vi "Switch status IO - Human Readable.vi"(1 "Switch status":path=path "C:/LabView/PPMS basic VIs/Switch Status.txt") -> (0 "String":string)   [LabVIEW 2016, in "pickering.lvclass"]
uses:
  pickering.lvclass
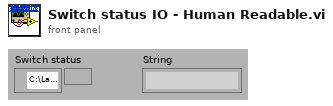
[diagram p1: front panel]
types:
  T1 = typedef "pickering.lvclass/Channels-Array.ctl" = T2[]
  T2 = typedef "pickering.lvclass/Channel-Cluster.ctl" = cluster{"Channel x":T3, "Channel y":T4}
  T3 = typedef "pickering.lvclass/ChannelX-ComboBox.ctl" = string
  T4 = typedef "pickering.lvclass/ChannelY-ComboBox.ctl" = string
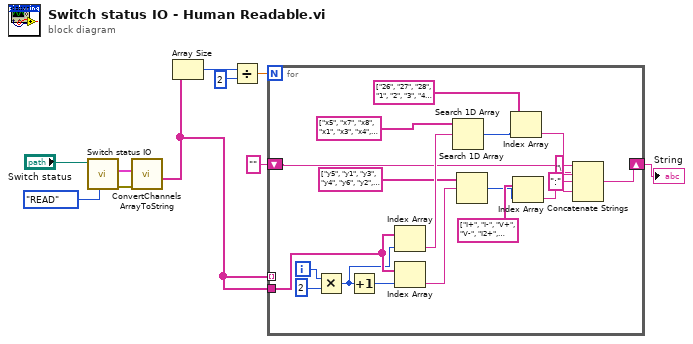
[diagram p0: block diagram]
diagram:
  n1 = call "Switch status IO.vi"("mode"=enum16{"READ", "WRITE"}."READ", "Path"="Switch status") -> ("error out"=w3:errorcluster, "Channels out"=w2:T1)  [unwired: 7 in, 1 out]
  n2 = call "ConvertChannelsArrayToString.vi"("error in (no error)"=w3, "Channels in"=w2) -> ("String array"=w1:string[])  [unwired: 7 in, 2 out]
  n3 = Array Size(array=w1) -> (size(s)=w6:i32)
  n4 = Divide(x=w6, y=2) -> (x/y=w8:dbl)
  n5 = for {
    N: w8 -> [_]
    tunnel: w1 -> [w29]
    tunnel: w1 -> [_] mode=indexing
    shift-right: [w16] -> w10
    shift-left: "" -> [w15]
    i -> [w27]
    n6 = Multiply(x=w27, y=2) -> (x*y=w25:i32)
    n7 = Increment(x=w25) -> (x+1=w28:i32)
    n8 = Index Array(array=w29, index=w25) -> (element=w23:string)
    n9 = Index Array(array=w29, index=w28) -> (element=w19:string)
    n10 = Search 1D Array(1D array=string[] ["x5", "x7", "x8", "x1", "x3", "x4", "x2", "x6"], element=w23) -> (index of element=w21:i32)  [unwired: 1 in]
    n11 = Search 1D Array(1D array=string[] ["y5", "y1", "y3", "y4", "y6", "y2", "y7", "y8"], element=w19) -> (index of element=w17:i32)  [unwired: 1 in]
    n12 = Index Array(array=string[] ["26", "27", "28", "1", "2", "3", "4", "5"], index=w21) -> (element=w12:string)
    n13 = Index Array(array=string[] ["I+", "I-", "V+", "V-", "I2+", "I2-", "V2+", "V2-"], index=w17) -> (element=w14:string)
    n14 = Concatenate Strings(w15, w14, ":" ("string"), w12, "\n" ("string")) -> (w16:string)
  }
  "String" <- w10
